vi "parse Header name (Channels).vi"(11 "EEG Single Channel":T1) -> (3 "String":string)   [LabVIEW 2016, in "Logger.lvlib"]
uses:
  Logger.lvlib
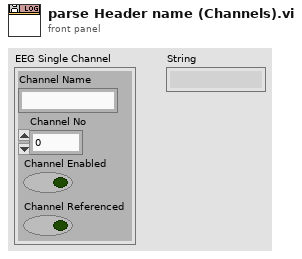
[diagram p1: front panel]
types:
  T1 = cluster{"Channel Name":string, "Channel No":u8, "Channel Enabled":bool, "Channel Referenced":bool}
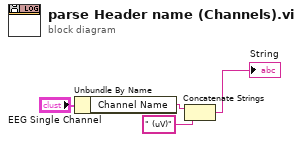
[diagram p0: block diagram]
diagram:
  n1 = Unbundle By Name("EEG Single Channel") -> ("Channel Name"=w2:string)
  n2 = Concatenate Strings(w2, " (uV)" ("string")) -> (→"String":string)
